vi "Element to Message Element Metadata.vi"(6 "repeated":bool, 8 "error in":errorcluster, 9 "protobuf index":i32, 10 "message element type":T2, 11 "message name":string) -> (0 "error out":errorcluster, 1 "element metadata":T1, 2 "nested cluster":bool)   [LabVIEW 2019, in "grpc-lvsupport.lvlib"]
uses:
  grpc-lvsupport.lvlib
  typeDefs/Message Element Type.ctl
  typeDefs/Message Element Metadata.ctl
  Shared/Well Known Types.ctl
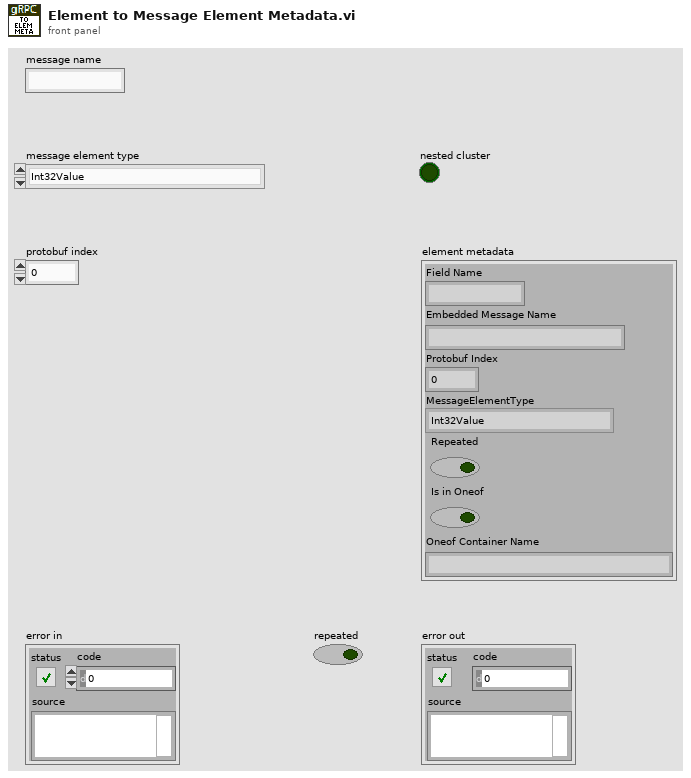
[diagram p1: front panel]
types:
  T1 = typedef "grpc-lvsupport.lvlib/Message Element Metadata.ctl" = cluster{"Field Name":string, "Embedded Message Name":string, "Protobuf Index":i32, "MessageElementType":T2, "Repeated":bool, "Is in Oneof":bool, "Oneof Container Name":string}
  T2 = typedef "grpc-lvsupport.lvlib/Message Element Type.ctl" = enum32{"Int32Value", "FloatValue", "DoubleValue", "BoolValue", "StringValue", "MessageValue", "Int64Value", "UInt32Value", "UInt64Value", "EnumValue", "Bytes", "Fixed64", "Fixed32", "SFixed64", "SFixed32", "SInt64", "SInt32"}
  T3 = typedef "grpc-lvsupport.lvlib/Well Known Types.ctl" = enum32{"None", "Double2DArray", "String2DArray"}
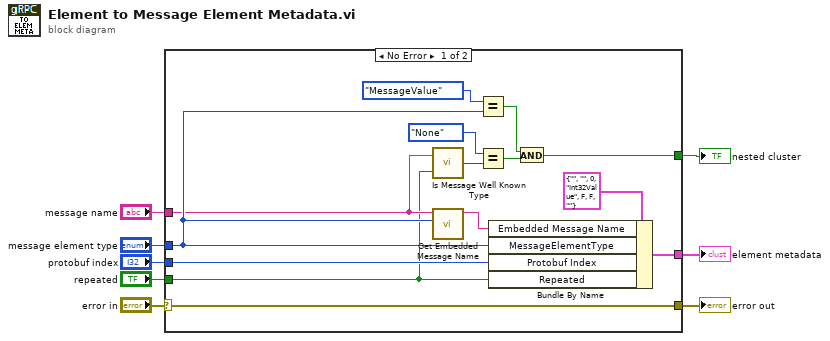
[diagram p0: block diagram]
diagram:
  n1 = case shown="No Error" "error in" {
    selector: "error in" -> [w16 w23]
    tunnel: "message element type" -> [w22 _]
    tunnel: "message name" -> [w15 _]
    tunnel: "protobuf index" -> [w21 _]
    tunnel: "repeated" -> [w14 _]
    tunnel: [w9 _] -> w4
    tunnel: [w20 _] -> w3
    tunnel: [w16 w23] -> w1
    frame No Error {
      n2 = call "Is Message Well Known Type.vi"("repeated"=w14, "message name"=w15) -> ("well known type"=w13:T3)
      n3 = call "Get Embedded Message Name.vi"("MessageElementType"=w22, "Element Name"=w15) -> ("Embedded Message Name"=w18:string)  [unwired: 9 in]
      n4 = Equal?(x=Message_Element_Type."MessageValue", y=w22) -> (x = y?=w10:bool)
      n5 = Equal?(x=Well_Known_Types."None", y=w13) -> (x = y?=w11:bool)
      n6 = Bundle By Name(cluster=T1 {"Field Name"="", "Embedded Message Name"="", "Protobuf Index"=0, "MessageElementType"=enum."Int32Value", "Repeated"=FALSE, "Is in Oneof"=FALSE, "Oneof Container Name"=""} ("MessageElementMetadata"), "Embedded Message Name"=w18, "MessageElementType"=w22, "Protobuf Index"=w21, "Repeated"=w14) -> (w20:T1)
      n7 = And(x=w10, y=w11) -> (x .and. y?=w9:bool)
    }
    frame Error {
    }
  }
  "nested cluster" <- w4
  "element metadata" <- w3
  "error out" <- w1
